vi "Set REF Phase to Zero.vi"(8 "error in (no error)":errorcluster, 9 "Reset Phase":bool, 11 "Instrument.DAQ":refnum<class "Instrument.DAQ.lvclass">) -> (0 "error out":errorcluster, 3 "Instrument.DAQ out":refnum<class "Instrument.DAQ.lvclass">)   [LabVIEW 2019, in "Instrument.Lockin.lvlib" / "Instrument.DAQ.lvclass"]
uses:
  Instrument.DAQ.lvclass
  Instrument.DAQ.lvclass/Instrument.DAQ.ctl
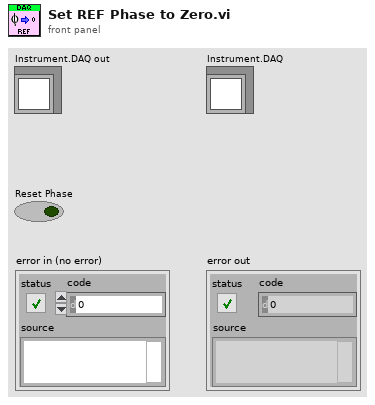
[diagram p1: front panel]
types:
  T1 = typedef "Instrument.Lockin.lvlib/Instrument.DAQ.lvclass/REF.Channel--Cluster--Array.ctl" = T2[]
  T2 = typedef "Instrument.Lockin.lvlib/Instrument.DAQ.lvclass/REF.Channel--Cluster.ctl" = cluster{"Enable?":bool, "Channel":i32, "Frequency":dbl, "Phase":dbl, "TC":dbl, "Roll-Off":i32}
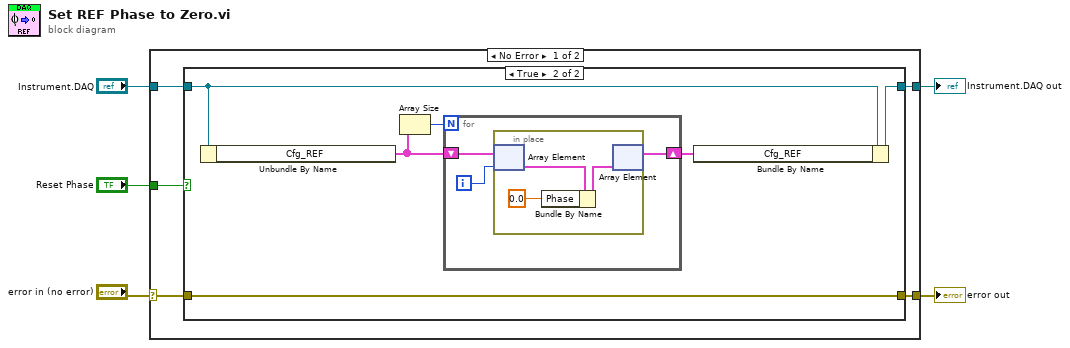
[diagram p0: block diagram]
diagram:
  n1 = case shown="No Error" "error in (no error)" {
    selector: "error in (no error)" -> [w7 w26]
    tunnel: "Instrument.DAQ" -> [w10 w25]
    tunnel: [w9 w25] -> w4
    tunnel: [w6 w26] -> w2
    tunnel: "Reset Phase" -> [w8 _]
    frame No Error {
      n2 = case shown="True" w8 {
        tunnel: w10 -> [w12 w18]
        tunnel: [w12 w17] -> w9
        tunnel: w7 -> [w11 w15]
        tunnel: [w11 w15] -> w6
        frame False {
        }
        frame True {
          n3 = Unbundle By Name(w18) -> ("Cfg_REF"=w13:T1)
          n4 = Array Size(array=w13) -> (size(s)=w14:i32)
          n5 = for {
            N: w14 -> [_]
            shift-right: [w20] -> w16
            shift-left: w13 -> [w21]
            i -> [w19]
            n6 = in-place {
              n7 = in-place-array #1(w21, w19) -> (w23:T2)
              n8 = Bundle By Name(cluster=w23, "Phase"=0.0) -> (w22:T2)
              n9 = in-place-array #1(w22) -> (w20:T1)  [unwired: 1 out]
            }
          }
          n10 = Bundle By Name(cluster=w18, "Cfg_REF"=w16) -> (w17:refnum<class "Instrument.DAQ.lvclass">)
        }
      }
    }
    frame Error {
    }
  }
  "Instrument.DAQ out" <- w4
  "error out" <- w2
